vi "Arm Limits.vi"(1 "Motor Input":dbl=-0.5, 2 "Current Angle":dbl=155.84632089769002) -> (0 "Motor Output":dbl=-0.5)   [LabVIEW 2013]
uses:
  Robot Global Data.vi
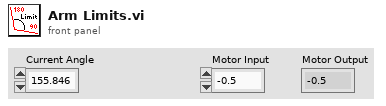
[diagram p1: front panel]
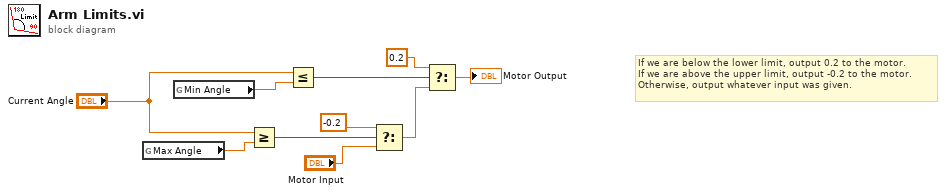
[diagram p0: block diagram]
diagram:
  # "If we are below the lower limit, output 0.2 to the motor.\nIf we are above the upper limit, output -0.2 to the motor.\nOtherwise, output whatever input was given."
  n1 = global read "Robot Global Data.vi" "Max Angle"() -> (w2:dbl)
  n2 = global read "Robot Global Data.vi" "Min Angle"() -> (w1:dbl)
  n3 = Greater Or Equal?(x="Current Angle", y=w2) -> (x >= y?=w9:bool)
  n4 = Less Or Equal?(x="Current Angle", y=w1) -> (x <= y?=w6:bool)
  n5 = Select(t=-0.2, s=w9, f="Motor Input") -> (s? t:f=w8:dbl)
  n6 = Select(t=0.2, s=w6, f=w8) -> (s? t:f=→"Motor Output":dbl)
